vi "Init.vi"(8 "error in (no error)":errorcluster, 10 "UI Options":T1, 11 "Cmd Q":refnum<queue>) -> (0 "error out":errorcluster)   [LabVIEW 2024, in "FormulaG.lvlib" / "UI Options Cmd.lvclass"]
uses:
  UI Options Cmd.lvclass
  FormulaG-Common/UI Options.ctl
  Command/Command.lvclass
  C:/dev/SummerOfLabVIEW/sol-formulag/Scorer 2024/FormulaG/Command/Command.lvclass
  UI Options Cmd.lvclass/UI Options Cmd.ctl
  FormulaG-Common/FormulaG-Common.lvlib
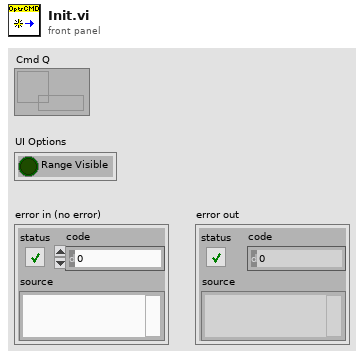
[diagram p1: front panel]
types:
  T1 = typedef "FormulaG-Common.lvlib/UI Options.ctl" = cluster{"Range Visible":bool}
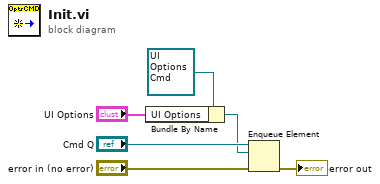
[diagram p0: block diagram]
diagram:
  n1 = Bundle By Name(cluster=refnum<class "UI Options Cmd.lvclass"> refnum ("FormulaG.lvlib:UI Options Cmd.lvclass"), "UI Options"="UI Options") -> (w1:refnum<class "UI Options Cmd.lvclass">)
  n2 = Enqueue Element(queue="Cmd Q", element=w1, error in (no error)="error in (no error)") -> (error out=→"error out":errorcluster)  [unwired: 1 in, 2 out]
